vi "Msg Receive.vi"(11 "Msg Receive in":refnum<class "Msg Receive.lvclass">) -> (0 "error out":errorcluster, 1 "Destroyed Self?":bool, 3 "Msg Receive out":refnum<class "Msg Receive.lvclass">)   [LabVIEW 2021, in "LVCAM.lvlib" / "Msg Receive.lvclass"]
uses:
  Msg Receive.lvclass
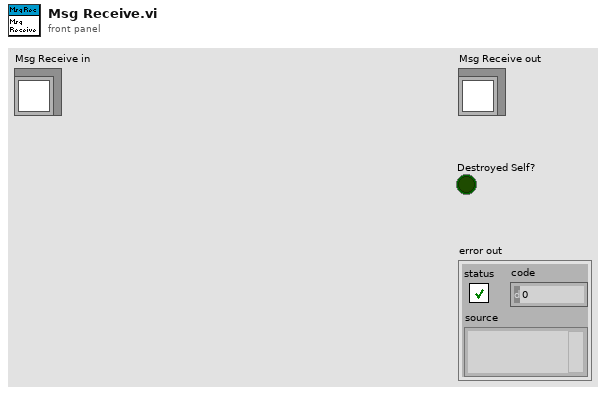
[diagram p1: front panel]
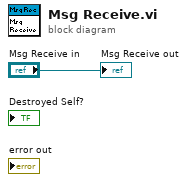
[diagram p0: block diagram]
diagram:
  "Msg Receive out" <- "Msg Receive in"
